vi "OE1022D_Configure Trigger.vi"(1 "Trigger Source (0: Internal)":u16(ring) items=["Internal", "External"], 3 "error in (no error)   2":errorcluster, 4 "OE1022D A/B":u8(ring) items=["Channel A", "Channel B"], 5 "VISA resource name   2":refnum<visa-resource-name>) -> (0 "error out   2":errorcluster, 2 "VISA resource name out   2":refnum<visa-resource-name>)   [LabVIEW 2022 SP3]
doc: "Configures the reference source and the internal oscillator."
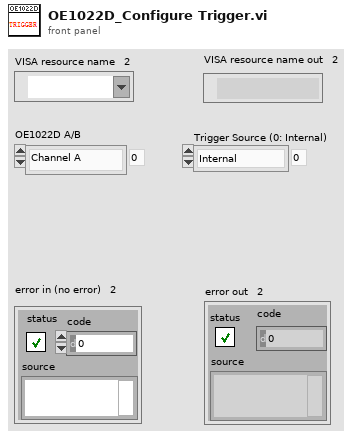
[diagram p1: front panel]
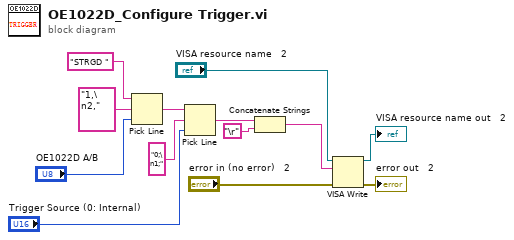
[diagram p0: block diagram]
diagram:
  n1 = Pick Line(string ("")="STRGD ", multi-line string="1,\n2,", line index="OE1022D A/B") -> (output string=w13:string)
  n2 = Pick Line(string ("")=w13, multi-line string="0;\n1;", line index="Trigger Source (0: Internal)") -> (output string=w4:string)
  n3 = Concatenate Strings(w4, "\r") -> (w3:string)
  n4 = VISA Write(VISA resource name="VISA resource name   2", write buffer=w3, error in (no error)="error in (no error)   2") -> (VISA resource name out=→"VISA resource name out   2":refnum<visa-resource-name>, error out=→"error out   2":errorcluster)  [unwired: 1 out]
